vi "Active Cell Position Separator.vi"(8 "error in (no error)":errorcluster, 10 "Boolean":bool, 11 "MCLB in":refnum<class "MulticolumnListbox.lvclass">) -> (0 "error out":errorcluster, 3 "MCLB out":refnum<class "MulticolumnListbox.lvclass">)   [LabVIEW 2023, in "MulticolumnListbox.lvclass"]
uses:
  MulticolumnListbox.lvclass
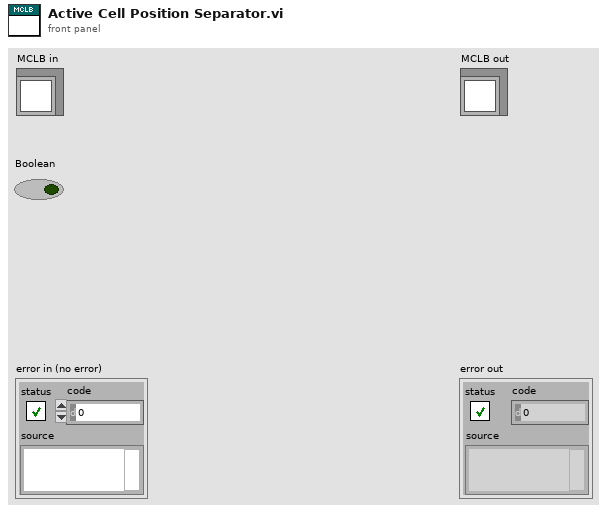
[diagram p1: front panel]
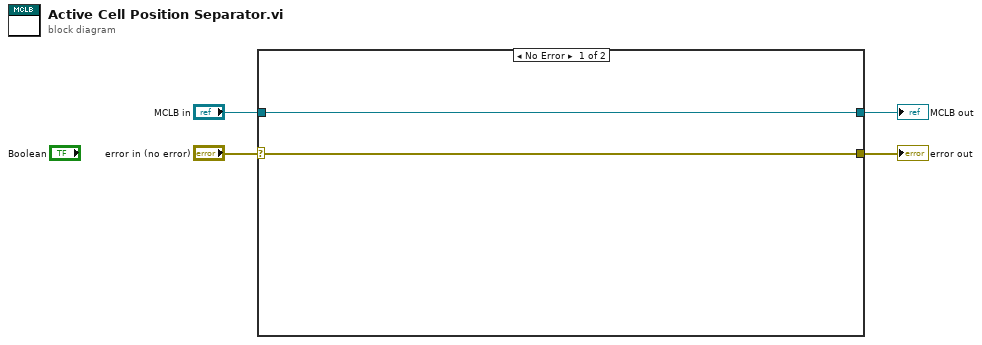
[diagram p0: block diagram]
diagram:
  n1 = case shown="No Error" "error in (no error)" {
    selector: "error in (no error)" -> [w5 w8]
    tunnel: [w5 w8] -> w3
    tunnel: [w6 w7] -> w1
    tunnel: "MCLB in" -> [w6 w7]
    frame No Error {
    }
    frame Error {
    }
  }
  "error out" <- w3
  "MCLB out" <- w1
